vi "Thermometer.vi"(1 "单位（0：摄氏度）":u16(ring) items=["摄氏度", "华氏度"]) -> (0 "温度":dbl(slide) scale=0.0..100.0)   [LabVIEW 2012]
doc: "本VI使用DAQ BNC-2120接线盒的温度传感器测量温度。"
uses:
  Instance           2 19Saved   Thermometer .vi
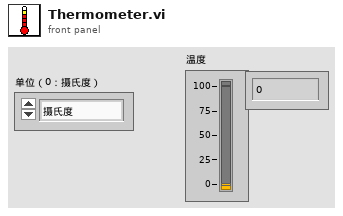
[diagram p1: front panel]
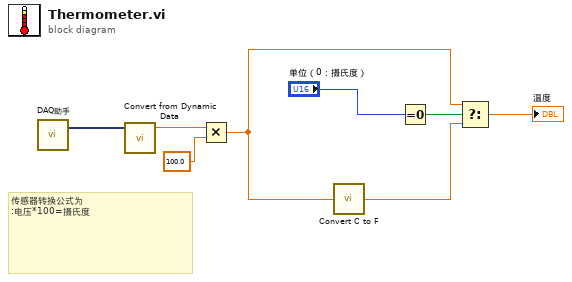
[diagram p0: block diagram]
diagram:
  # "传感器转换公式为\n:电压*100=摄氏度"
  n1 = call "DAQ助手"() -> ("data"=w1:dynamicdata)  [unwired: 17 in, 2 out]
  n2 = call "Convert from Dynamic Data"("Dynamic Data Type"=w1) -> ("Scalar"=w6:dbl)  [unwired: 3 in]
  n3 = Multiply ("乘")(x=w6, y=100.0) -> (x*y=w7:dbl)
  n4 = call "Convert C to F.vi"("摄氏温标"=w7) -> ("华氏温标"=w8:dbl)
  n5 = Equal To 0? ("等于0？")(x="单位（0：摄氏度）") -> (x = 0?=w2:bool)
  n6 = Select ("选择")(t=w7, s=w2, f=w8) -> (s? t:f=→"温度":dbl)
